vi "ScalingFactorProperty.vi"(7 "Write?":bool, 8 "error in (no error)":errorcluster, 10 "Value in":dbl, 11 "QRCodeDetector in":refnum<class "QRDetector.lvclass">) -> (0 "error out":errorcluster, 3 "Value out":dbl)   [LabVIEW 2020, in "g_ar_toolkit.feature_detection.lvlib" / "QRDetector.lvclass"]
uses:
  QRDetector.lvclass
  QRDetector.lvclass/QRDetector.ctl
  g_ar_toolkit.common/g_ar_toolkit.common.lvlib
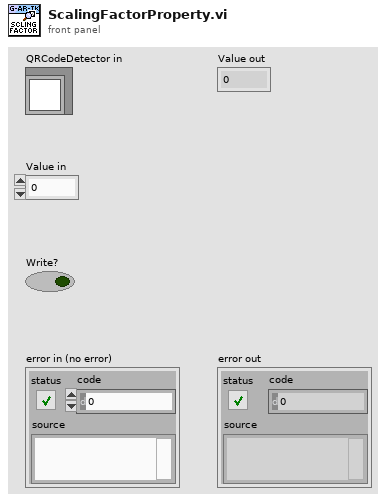
[diagram p1: front panel]
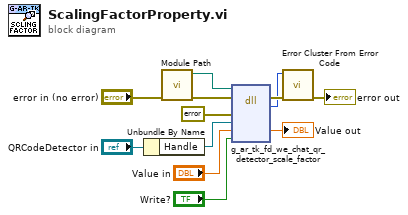
[diagram p0: block diagram]
diagram:
  n1 = Unbundle By Name("QRCodeDetector in") -> ("Handle"=w8:refnum<data-value>)
  n2 = call "Module Path.vi"("error in (no error)"="error in (no error)") -> ("error out"=w2:errorcluster, "Path"=w1:path)  [unwired: 9 in]
  n3 = dll-call lib="?" fn="g_ar_tk_fd_we_chat_qr_detector_scale_factor" ("g_ar_toolkit.*.*:g_ar_tk_capture_context_create")(path in=w1, error in=w2, "error_cluster"=errorcluster {"status"=FALSE, "code"=0, "source"=""} ("error constant"), "Detector_EDVR"=w8, "Value"="Value in", "Write"="Write?") -> (error out=w5:errorcluster, "MgErr"=w4:i32, "Value"=→"Value out":dbl)  [unwired: 4 in, 1 out]
  n4 = call <vilib>:"Error Cluster From Error Code.vi"("error in (no error)"=w5, "error code (0)"=w4) -> ("error out"=→"error out":errorcluster)  [unwired: 7 in]
